vi "SerializeObject.vi"(8 "error in (no error)":errorcluster, 9 "Pretty Print?":bool=TRUE, 11 "ViPER_Base in":refnum<class "ViPER.lvclass">) -> (0 "error out":errorcluster, 2 "Object XML":string, 3 "ViPER_Base out":refnum<class "ViPER.lvclass">)   [LabVIEW 2022 SP3, in "ViPER.lvlib" / "ViPER.lvclass"]
uses:
  ViPER.lvclass
  <vilib>/xml/Load XML String.vi
  <vilib>/xml/Close Reference(Node).vi
  <vilib>/xml/NI_XML.lvlib
  <resource>/objmgr/DOMUserDefRef.rc
panel:
  # "### BSD License (http://www.opensource.org/licenses/bsd-license.php) Begin ###\n\nCopyright (c) 2018  Kurt Friday www.medulla.net\n\nAll rights reserved.\n\nRedistribution and use in source and binary forms, with or without\nmodification, are permitted provided that the following conditions are met:\n\n    * Redistributions of source code must retain the above copyright\n      notice, this list of conditions and the following disclaimer.\n\n    * Redistributions in binary form must reproduce the above copyright\n      notice, this list of conditions and the following disclaimer in the\n      documentation and/or other materials provided with the distribution.\n\n    * Neither the name of the <organization> nor the\n      names of its contributors may be used to endorse or promote products\n      derived from this software without specific prior written permission.\n\nTHIS SOFTWARE IS PROVIDED BY THE COPYRIGHT HOLDERS AND CONTRIBUTORS \"AS IS\" AND\nANY EXPRESS OR IMPLIED WARRANTIES, INCLUDING, BUT NOT LIMITED TO, THE IMPLIED\nWARRANTIES OF MERCHANTABILITY AND FITNESS FOR A PARTICULAR PURPOSE ARE\nDISCLAIMED. IN NO EVENT SHALL <COPYRIGHT HOLDER> BE LIABLE FOR ANY\nDIRECT, INDIRECT, INCIDENTAL, SPECIAL, EXEMPLARY, OR CONSEQUENTIAL DAMAGES\n(INCLUDING, BUT NOT LIMITED TO, PROCUREMENT OF SUBSTITUTE GOODS OR SERVICES;\nLOSS OF USE, DATA, OR PROFITS; OR BUSINESS INTERRUPTION) HOWEVER CAUSED AND\nON ANY THEORY OF LIABILITY, WHETHER IN CONTRACT, STRICT LIABILITY, OR TORT\n(INCLUDING NEGLIGENCE OR OTHERWISE) ARISING IN ANY WAY OUT OF THE USE OF THIS\nSOFTWARE, EVEN IF ADVISED OF THE POSSIBILITY OF SUCH DAMAGE."
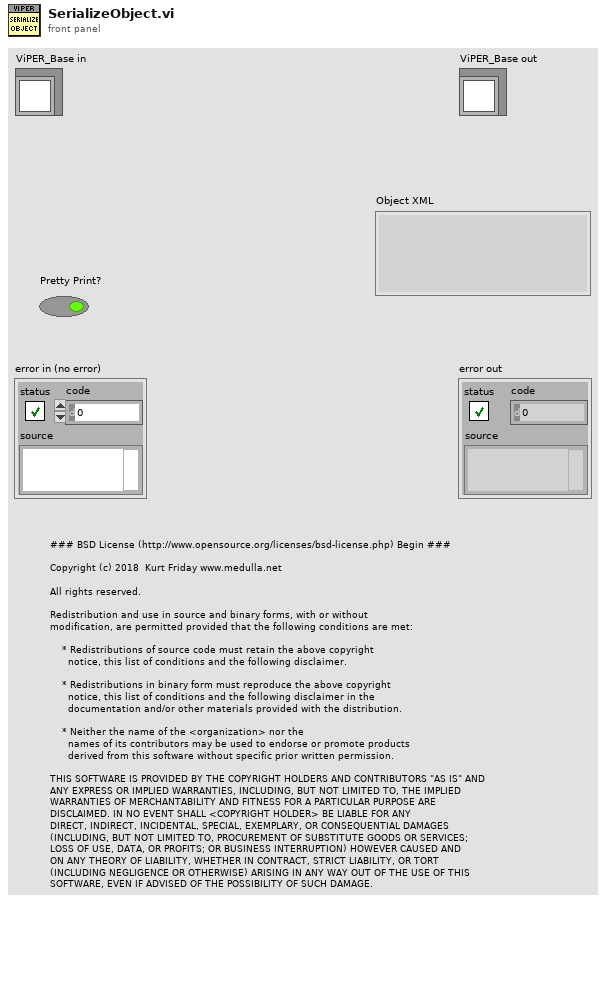
[diagram p1: front panel]
types:
  T1 = typedef "ViPER.lvlib/ViPER.lvclass/ObjectAttributes.ctl" = cluster{"Object":T2, "Ancestors":T4[], "Config":T5, "Init_OK":bool, "Hierachy":string[], "PPL?":bool[], "SFP_Open":bool[], "Config_SFP_Open":bool[], "SoftFP_event":refnum<user-event>[], "ConfigFP_event":refnum<user-event>[], "SoftFP_Shutdown_Notifier":refnum<notifier>[], "ConfigFP_Shutdown_Notifier":refnum<notifier>[]}
  T2 = typedef "ViPER.lvlib/ViPER.lvclass/ObjectDefinition.ctl" = cluster{"Name":string, "Ancestors":T3[]}
  T3 = typedef "ViPER.lvlib/ViPER.lvclass/Ancestor.ctl" = cluster{"Class":string, "Config":string, "Objects":string[]}
  T4 = typedef "ViPER.lvlib/ViPER.lvclass/ObjectLayers.ctl" = cluster{"Ancestor":string, "Objects":refnum<class "ViPER.lvclass">[], "Object_Names":string[], "Owned":bool[]}
  T5 = typedef "ViPER.lvlib/ViPER.lvclass/Config.ctl" = cluster{"default":string}
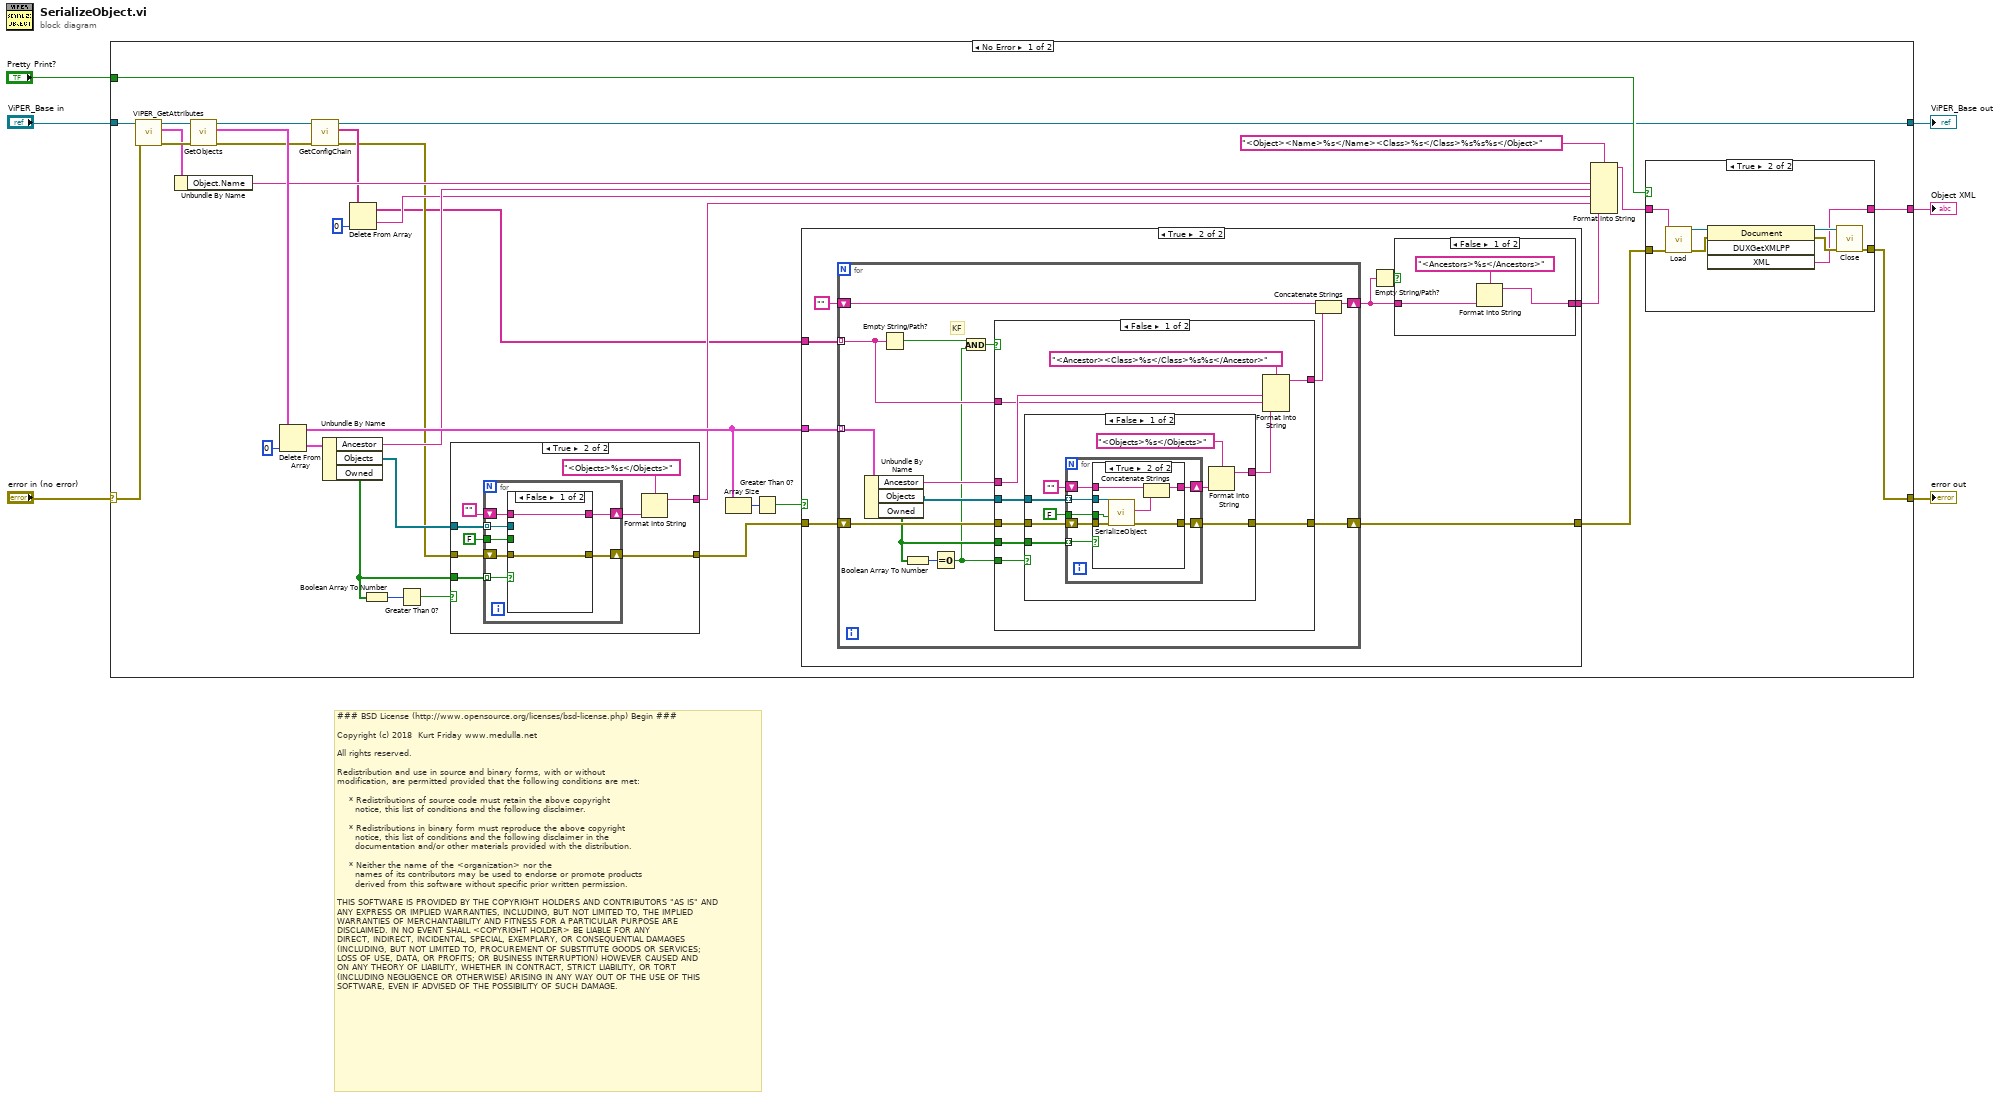
[diagram p0: block diagram]
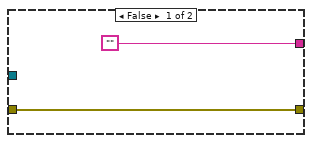
[diagram p3: hidden frame]
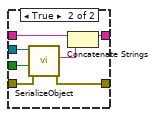
[diagram p4: hidden frame]
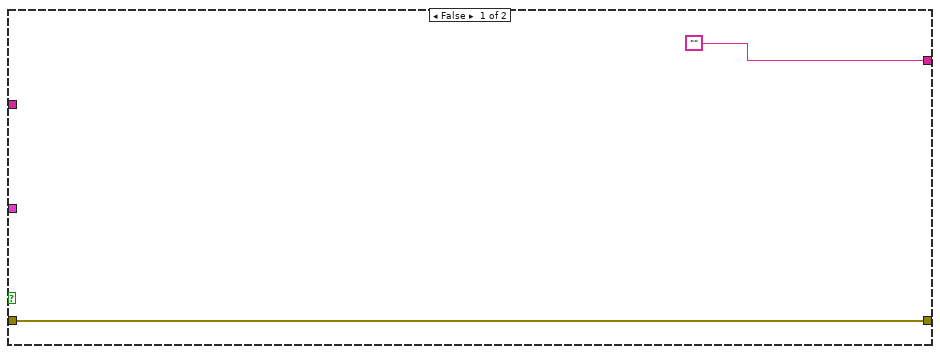
[diagram p5: hidden frame]
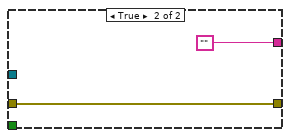
[diagram p8: hidden frame]
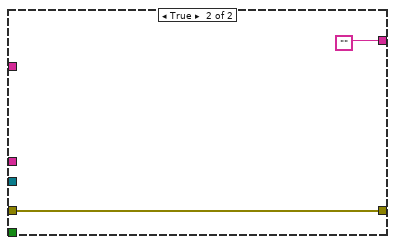
[diagram p9: hidden frame]
diagram:
  # "### BSD License (http://www.opensource.org/licenses/bsd-license.php) Begin ###\n\nCopyright (c) 2018  Kurt Friday www.medulla.net\n\nAll rights reserved.\n\nRedistribution and use in source and binary forms, with or without\nmodification, are permitted provided that the following conditions are met:\n\n    * Redistributions of source code must retain the above copyright\n      notice, this list of conditions and the following disclaimer.\n\n    * Redistributions in binary form must reproduce the above copyright\n      notice, this list of conditions and the following disclaimer in the\n      documentation and/or other materials provided with the distribution.\n\n    * Neither the name of the <organization> nor the\n      names of its contributors may be used to endorse or promote products\n      derived from this software without specific prior written permission.\n\nTHIS SOFTWARE IS PROVIDED BY THE COPYRIGHT HOLDERS AND CONTRIBUTORS \"AS IS\" AND\nANY EXPRESS OR IMPLIED WARRANTIES, INCLUDING, BUT NOT LIMITED TO, THE IMPLIED\nWARRANTIES OF MERCHANTABILITY AND FITNESS FOR A PARTICULAR PURPOSE ARE\nDISCLAIMED. IN NO EVENT SHALL <COPYRIGHT HOLDER> BE LIABLE FOR ANY\nDIRECT, INDIRECT, INCIDENTAL, SPECIAL, EXEMPLARY, OR CONSEQUENTIAL DAMAGES\n(INCLUDING, BUT NOT LIMITED TO, PROCUREMENT OF SUBSTITUTE GOODS OR SERVICES;\nLOSS OF USE, DATA, OR PROFITS; OR BUSINESS INTERRUPTION) HOWEVER CAUSED AND\nON ANY THEORY OF LIABILITY, WHETHER IN CONTRACT, STRICT LIABILITY, OR TORT\n(INCLUDING NEGLIGENCE OR OTHERWISE) ARISING IN ANY WAY OUT OF THE USE OF THIS\nSOFTWARE, EVEN IF ADVISED OF THE POSSIBILITY OF SUCH DAMAGE."
  n1 = case shown="No Error" "error in (no error)" {
    selector: "error in (no error)" -> [w39 w146]
    tunnel: [w21 w146] -> w5
    tunnel: [w8 w145] -> w3
    tunnel: "ViPER_Base in" -> [w40 w145]
    tunnel: [w19 _] -> w2
    tunnel: "Pretty Print?" -> [w18 _]
    frame No Error {
      n2 = call "ViPER_GetAttributes.vi"("error in (no error)"=w39, "reference in"=w40) -> ("error out"=w37:errorcluster, "Data"=w28:T1, "reference out"=w38:refnum<class "ViPER.lvclass">)  [unwired: 6 in, 1 out]
      n3 = Unbundle By Name(w28) -> ("Object.Name"=w27:string)
      n4 = call "GetObjects.vi"("error in (no error)"=w37, "reference in"=w38) -> ("error out"=w30:errorcluster, "Ancestors"=w36:T4[], "reference out"=w31:refnum<class "ViPER.lvclass">)  [unwired: 7 in]
      n5 = Delete From Array(array=w36, index=0) -> (deleted portion=w29:T4, array with subset deleted=w35:T4[])  [unwired: 1 in]
      n6 = call-dynamic "GetConfigChain.vi"("error in (no error)"=w30, "reference in"=w31) -> ("error out"=w9:errorcluster, "Config out"=w10:string[], "reference out"=w8:refnum<class "ViPER.lvclass">)  [unwired: 7 in]
      n7 = Unbundle By Name(w29) -> ("Ancestor"=w26:string, "Objects"=w25:refnum<class "ViPER.lvclass">[], "Owned"=w11:bool[])
      n8 = Delete From Array(array=w10, index=0) -> (deleted portion=w17:string, array with subset deleted=w7:string[])  [unwired: 1 in]
      n9 = Boolean Array To Number(Boolean array=w11) -> (number=w13:u32)
      n10 = Greater Than 0?(x=w13) -> (x > 0?=w12:bool)
      n11 = case shown="True" w12 {
        tunnel: w25 -> [_ w61]
        tunnel: w9 -> [w51 w60]
        tunnel: ["" w56] -> w24
        tunnel: [w51 w54] -> w14
        tunnel: w11 -> [_ w53]
        frame False {
        }
        frame True {
          n12 = for {
            tunnel: w61 -> [w68] mode=indexing
            shift-right: [w66] -> w54
            shift-left: w60 -> [w67]
            shift-right: [w64] -> w58
            shift-left: "" -> [w65]
            tunnel: FALSE ("Pretty Print?") -> [w63]
            tunnel: w53 -> [w62] mode=indexing
            n13 = case shown="False" w62 {
              tunnel: w68 -> [_ w77]
              tunnel: w67 -> [w69 w76]
              tunnel: [w69 w75] -> w66
              tunnel: w65 -> [w70 w74]
              tunnel: [w70 w72] -> w64
              tunnel: w63 -> [_ w71]
              frame False {
              }
              frame True {
                n14 = call-dynamic "SerializeObject.vi"("error in (no error)"=w76, "Pretty Print?"=w71, "ViPER_Base in"=w77) -> ("error out"=w75:errorcluster, "Object XML"=w73:string)  [unwired: 6 in, 1 out]
                n15 = Concatenate Strings(w74, w73) -> (w72:string)
              }
            }
          }
          n16 = Format Into String(format string="<Objects>%s</Objects>", w58) -> (resulting string=w56:string)  [unwired: 2 in, 1 out]
        }
      }
      n17 = Array Size(array=w35) -> (size(s)=w34:i32)
      n18 = Greater Than 0?(x=w34) -> (x > 0?=w33:bool)
      n19 = case shown="True" w33 {
        tunnel: w14 -> [w79 w87]
        tunnel: [w79 w86] -> w22
        tunnel: w35 -> [_ w85]
        tunnel: ["" w83] -> w23
        tunnel: w7 -> [_ w82]
        frame False {
        }
        frame True {
          n20 = for {
            tunnel: w85 -> [w105] mode=indexing
            shift-right: [w103] -> w86
            shift-left: w87 -> [w104]
            shift-right: [w99] -> w81
            shift-left: "" -> [w98]
            tunnel: w82 -> [w94] mode=indexing
            # "KF"
            n21 = Unbundle By Name(w105) -> ("Ancestor"=w101:string, "Objects"=w102:refnum<class "ViPER.lvclass">[], "Owned"=w96:bool[])
            n22 = Empty String/Path?(string/path=w94) -> (empty?=w95:bool)
            n23 = Boolean Array To Number(Boolean array=w96) -> (number=w97:u32)
            n24 = Equal To 0?(x=w97) -> (x = 0?=w93:bool)
            n25 = And(x=w95, y=w93) -> (x .and. y?=w92:bool)
            n26 = case shown="False" w92 {
              tunnel: w104 -> [w115 w144]
              tunnel: [w114 w144] -> w103
              tunnel: w102 -> [w113 _]
              tunnel: w101 -> [w111 _]
              tunnel: [w109 ""] -> w100
              tunnel: w96 -> [w108 _]
              tunnel: w93 -> [w107 _]
              tunnel: w94 -> [w106 _]
              frame False {
                n27 = case shown="False" w107 {
                  tunnel: w115 -> [w124 w142]
                  tunnel: [w123 w142] -> w114
                  tunnel: w113 -> [w122 _]
                  tunnel: [w118 ""] -> w110
                  tunnel: w108 -> [w116 _]
                  frame False {
                    n28 = for {
                      tunnel: w122 -> [w131] mode=indexing
                      shift-right: [w129] -> w123
                      shift-left: w124 -> [w130]
                      shift-right: [w127] -> w120
                      shift-left: "" -> [w128]
                      tunnel: FALSE ("Pretty Print?") -> [w126]
                      tunnel: w116 -> [w125] mode=indexing
                      n29 = case shown="True" w125 {
                        tunnel: w131 -> [_ w140]
                        tunnel: w130 -> [w132 w139]
                        tunnel: [w132 w138] -> w129
                        tunnel: w128 -> [w133 w137]
                        tunnel: [w133 w135] -> w127
                        tunnel: w126 -> [_ w134]
                        frame False {
                        }
                        frame True {
                          n30 = call-dynamic "SerializeObject.vi"("error in (no error)"=w139, "Pretty Print?"=w134, "ViPER_Base in"=w140) -> ("error out"=w138:errorcluster, "Object XML"=w136:string)  [unwired: 6 in, 1 out]
                          n31 = Concatenate Strings(w137, w136) -> (w135:string)
                        }
                      }
                    }
                    n32 = Format Into String(format string="<Objects>%s</Objects>", w120) -> (resulting string=w118:string)  [unwired: 2 in, 1 out]
                  }
                  frame True {
                  }
                }
                n33 = Format Into String(format string="<Ancestor><Class>%s</Class>%s%s</Ancestor>", w111, w106, w110) -> (resulting string=w109:string)  [unwired: 2 in, 1 out]
              }
              frame True {
              }
            }
            n34 = Concatenate Strings(w98, w100) -> (w99:string)
          }
          n35 = Empty String/Path?(string/path=w81) -> (empty?=w80:bool)
          n36 = case shown="False" w80 {
            tunnel: [w89 w91] -> w83
            tunnel: w81 -> [w88 w91]
            frame False {
              n37 = Format Into String(format string="<Ancestors>%s</Ancestors>", w88) -> (resulting string=w89:string)  [unwired: 2 in, 1 out]
            }
            frame True {
            }
          }
        }
      }
      n38 = Format Into String(format string="<Object><Name>%s</Name><Class>%s</Class>%s%s%s</Object>", w27, w26, w17, w24, w23) -> (resulting string=w20:string)  [unwired: 2 in, 1 out]
      n39 = case shown="True" w18 {
        tunnel: w22 -> [w42 w50]
        tunnel: [w42 w45] -> w21
        tunnel: w20 -> [w41 w44]
        tunnel: [w41 w43] -> w19
        frame False {
        }
        frame True {
          n40 = call-poly <vilib>:"Load.vi"("XML string"=w44, "error in (no error)"=w50) -> ("DOM document out"=w49:refnum<k20>, "error out"=w46:errorcluster)  [unwired: 11 in, 1 out]
          n41 = invoke class="Document" method="DUXGetXMLPP"(reference=w49, error in=w46) -> (reference out=w48:refnum<k20>, error out=w47:errorcluster, "XML"=w43:string)  [unwired: 2 in, 1 out]
          n42 = call-poly <vilib>:"Close.vi"("error in (no error)"=w47, "node"=w48) -> ("error out"=w45:errorcluster)  [unwired: 7 in]
        }
      }
    }
    frame Error {
    }
  }
  "error out" <- w5
  "ViPER_Base out" <- w3
  "Object XML" <- w2
